vi "TrackerDLL.vi"() -> ()   [LabVIEW 2011]
panel:
  in  "tracker DLL path":path=path "cputrack.dll"
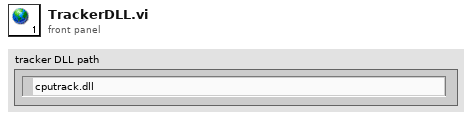
[diagram p1: front panel]
diagram:
